vi "Set Address Device.vi"(8 "error in (no error)":errorcluster, 10 "Device":string) -> (0 "error out":errorcluster, 3 "find list":string[](array[string]))   [LabVIEW 2015]
uses:
  <vilib>/Utility/file.llb/Read Delimited Spreadsheet (string).vi
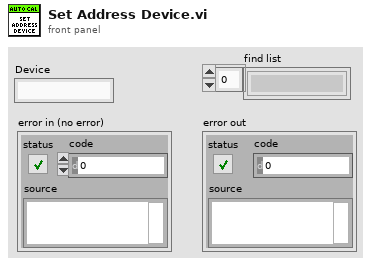
[diagram p1: front panel]
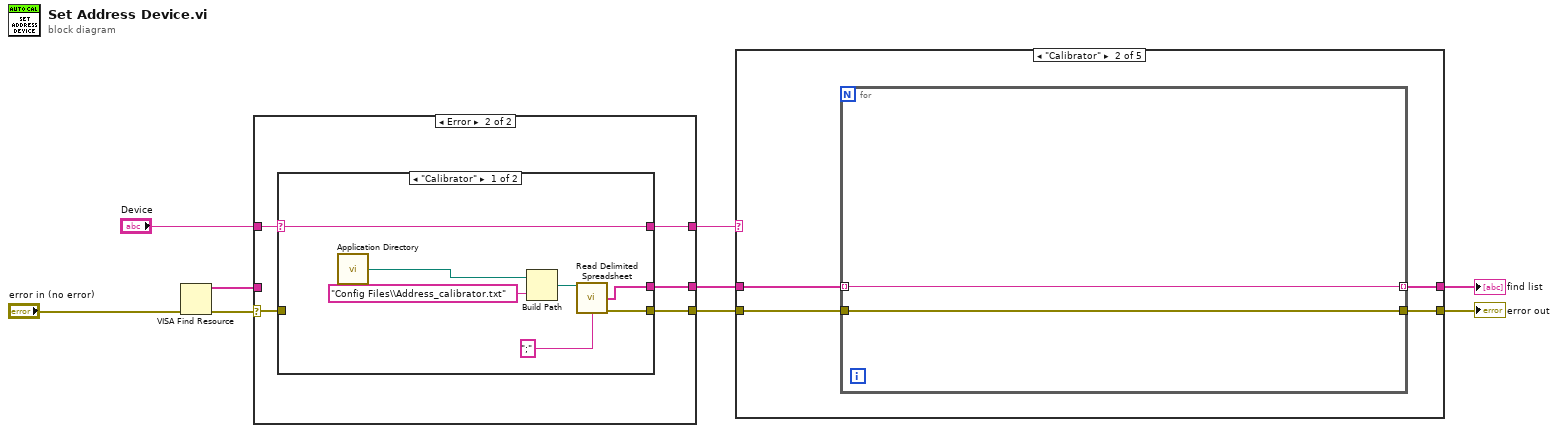
[diagram p0: block diagram]
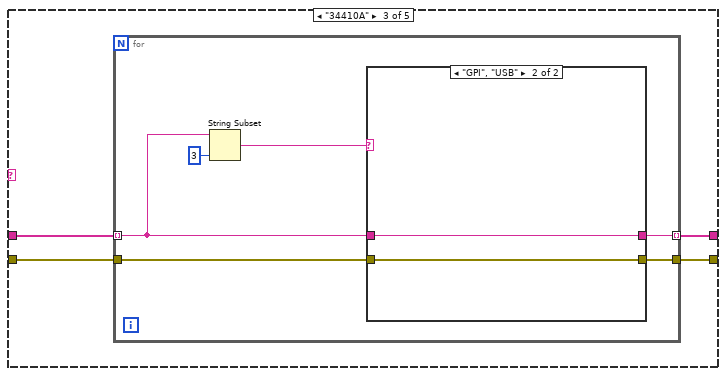
[diagram p3: hidden frame]
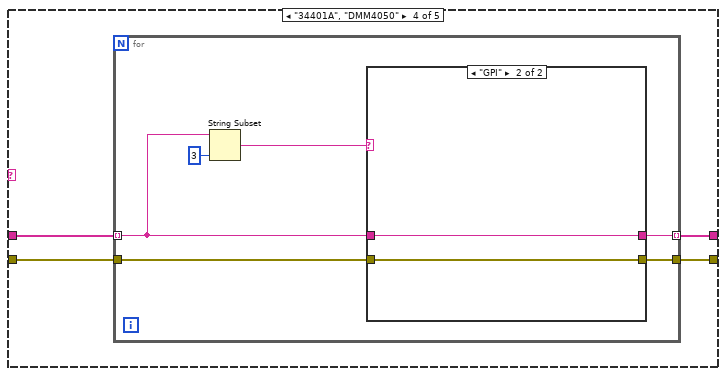
[diagram p5: hidden frame]
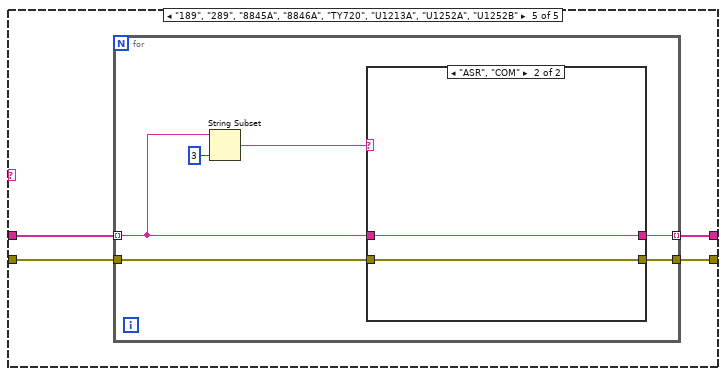
[diagram p7: hidden frame]
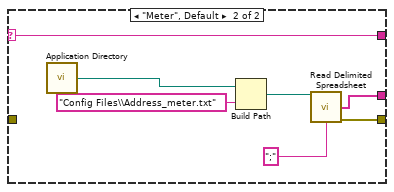
[diagram p10: hidden frame]
diagram:
  n1 = VISA Find Resource(8:"error in (no error)") -> (0:w8:errorcluster, 3:w7:string[])  [unwired: 2 in, 1 out]
  n2 = case shown="Error" w8 {
    selector: w8 -> [w11 w14]
    tunnel: [w12 w15] -> w5
    tunnel: w7 -> [w12 _]
    tunnel: [w11 w16] -> w4
    tunnel: "Device" -> [w10 w17]
    tunnel: [w10 w13] -> w3
    frame No Error {
    }
    frame Error {
      n3 = case shown="\"Calibrator\"" w17 {
        selector: w17 -> [w18 w25]
        tunnel: [w20 w27] -> w16
        tunnel: [w19 w28] -> w15
        tunnel: w14 -> [_ _]
        tunnel: [w18 w25] -> w13
        frame "Calibrator" {
          n4 = call <vilib>:"Application Directory.vi"() -> ("Application Directory"=w24:path)
          n5 = Build Path(base path=w24, name or relative path="Config Files\\Address_calibrator.txt") -> (appended path=w22:path)
          n6 = call-poly <vilib>:"Read Delimited Spreadsheet.vi"("file path (dialog if empty)"=w22, "delimiter (\\t)"=";" ("delimiter (\\t)")) -> ("first row"=w19:string[], "error out"=w20:errorcluster)  [unwired: 8 in, 4 out]
        }
        frame "Meter", Default {
          n7 = call <vilib>:"Application Directory.vi"() -> ("Application Directory"=w30:path)
          n8 = Build Path(base path=w30, name or relative path="Config Files\\Address_meter.txt") -> (appended path=w29:path)
          n9 = call-poly <vilib>:"Read Delimited Spreadsheet.vi"("file path (dialog if empty)"=w29, "delimiter (\\t)"=";" ("delimiter (\\t)")) -> ("first row"=w28:string[], "error out"=w27:errorcluster)  [unwired: 8 in, 4 out]
        }
      }
    }
  }
  n10 = case shown="\"Calibrator\"" w3 {
    tunnel: [w33 w35 w41 w54 w67] -> w2
    tunnel: w5 -> [w33 w37 w43 w56 w69]
    tunnel: [w32 w34 w40 w53 w66] -> w1
    tunnel: w4 -> [w32 w36 w42 w55 w68]
    frame "False", Default {
    }
    frame "Calibrator" {
      n11 = for {
        tunnel: w37 -> [w39] mode=indexing
        tunnel: w36 -> [w38]
        tunnel: [w39] -> w35 mode=indexing
        tunnel: [w38] -> w34
      }
    }
    frame "34410A" {
      n12 = for {
        tunnel: w43 -> [w48] mode=indexing
        tunnel: w42 -> [w45]
        tunnel: [w47] -> w41 mode=indexing
        tunnel: [w46] -> w40
        n13 = String Subset(string=w48, length (rest)=3 ("length (rest)")) -> (substring=w44:string)  [unwired: 1 in]
        n14 = case shown="\"GPI\", \"USB\"" w44 {
          tunnel: w48 -> [_ w52]
          tunnel: [_ w52] -> w47
          tunnel: [w50 w51] -> w46
          tunnel: w45 -> [w50 w51]
          frame "False", Default {
          }
          frame "GPI", "USB" {
          }
        }
      }
    }
    frame "34401A", "DMM4050" {
      n15 = for {
        tunnel: w56 -> [w61] mode=indexing
        tunnel: w55 -> [w58]
        tunnel: [w60] -> w54 mode=indexing
        tunnel: [w59] -> w53
        n16 = String Subset(string=w61, length (rest)=3 ("length (rest)")) -> (substring=w57:string)  [unwired: 1 in]
        n17 = case shown="\"GPI\"" w57 {
          tunnel: w61 -> [_ w65]
          tunnel: [_ w65] -> w60
          tunnel: [w63 w64] -> w59
          tunnel: w58 -> [w63 w64]
          frame "False", Default {
          }
          frame "GPI" {
          }
        }
      }
    }
    frame "189", "289", "8845A", "8846A", "TY720", "U1213A", "U1252A", "U1252B" {
      n18 = for {
        tunnel: w69 -> [w74] mode=indexing
        tunnel: w68 -> [w71]
        tunnel: [w73] -> w67 mode=indexing
        tunnel: [w72] -> w66
        n19 = String Subset(string=w74, length (rest)=3 ("length (rest)")) -> (substring=w70:string)  [unwired: 1 in]
        n20 = case shown="\"ASR\", \"COM\"" w70 {
          tunnel: w74 -> [_ w78]
          tunnel: [_ w78] -> w73
          tunnel: [w76 w77] -> w72
          tunnel: w71 -> [w76 w77]
          frame "False", Default {
          }
          frame "ASR", "COM" {
          }
        }
      }
    }
  }
  "find list" <- w2
  "error out" <- w1
